vi "M02 Toy Factory.vi"(11 "EV3 in":T1) -> (3 "NXT/EV3":T1)   [LabVIEW 2016]
uses:
  <vilib>/NXT/Subs/LVHSConnector.ctl
  <vilib>/NXT/LegoClasses/BrickReference/BrickReference.lvclass
  <vilib>/NXT/Block Support/NXT_OutputPort.ctl
  <vilib>/NXT/NXTIO Xnodes/NXTIONodeSubVIs/NXTMotorRunDistance.vi
  <vilib>/NXT/NXTIO Xnodes/AddressXNode/NXTIOAddress.xnode
  <vilib>/NXT/NXTIO Xnodes/NXTIOXNode/NXTIO.xnode
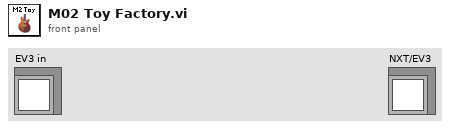
[diagram p1: front panel]
types:
  T1 = typedef "LVHSConnector.ctl" = refnum<class "BrickReference.lvclass">
  T2 = typedef "NXT_OutputPort.ctl" = u8
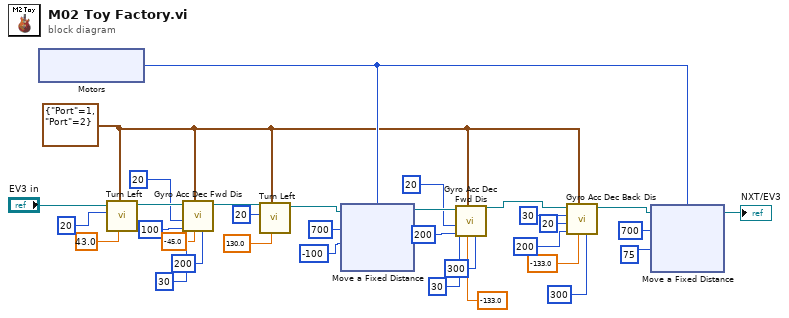
[diagram p0: block diagram]
diagram:
  w3 = cluster{"Port":T2, "Port":T2} {"Port"=1, "Port"=2} ("Motor")
  n1 = xnode "Motors"() -> ("Motor"=w4:T2)
  n2 = call "Turn Left.vi"("Turning angle"=sgl 43.0, "Motor"=w3, "Motor B (right)"=i8 20, "EV3 in"="EV3 in") -> ("EV3 out"=w11:T1)  [unwired: 7 in]
  n3 = call "Gyro Acc Dec Fwd Dis.vi"("Stop rotation"=200, "Ini. Degrees"=sgl -45.0, "Motor"=w3, "Threshold to De-acc"=100, "De-acc"=20, "Acc"=30, "EV3 in"=w11) -> ("EV3 out"=w13:T1)  [unwired: 4 in]
  n4 = call "Turn Left.vi"("Turning angle"=sgl 130.0, "Motor"=w3, "Motor B (right)"=i8 20, "EV3 in"=w13) -> ("EV3 out"=w17:T1)  [unwired: 7 in]
  n5 = xnode "Move a Fixed Distance"("Speed 1"=i8 -100, "Distance 1"=700, "Motors"=w4, "NXT/EV3"=w17) -> ("NXT/EV3"=w24:T1)
  n6 = call "Gyro Acc Dec Fwd Dis.vi"("Stop rotation"=300, "Ini. Degrees"=sgl -133.0, "Motor"=w3, "Threshold to De-acc"=200, "De-acc"=20, "Acc"=30, "EV3 in"=w24) -> ("EV3 out"=w30:T1)  [unwired: 4 in]
  n7 = call "Gyro Acc Dec Back Dis.vi"("Stop rotation"=300, "Ini. Degrees"=sgl -133.0, "Motor"=w3, "Threshold to De-acc"=200, "De-acc"=20, "Acc"=30, "EV3 in"=w30) -> ("EV3 out"=w33:T1)  [unwired: 4 in]
  n8 = xnode "Move a Fixed Distance"("Speed 1"=i8 75, "Distance 1"=700, "Motors"=w4, "NXT/EV3"=w33) -> ("NXT/EV3"=→"NXT/EV3":T1)
